vi "_Anritsu_SA_Write_Read.vi"(4 "bytes to read":i32=100, 6 "Comand":string="SNGLS\nSMA? 0,11", 7 "address":string="192.168.0.6") -> (0 "error out":errorcluster, 3 "Data out":i32[](array[numeric])=[-115184, -121571, -123353, -121687, -116570, -110499, -109976, -114455, -117677, -117596, -114322])   [LabVIEW 2013]
panel:
  out "data out":string="-115184,-121571,-123353,-121687,-116570,-110499,-109976,-114455,-117677,-117596,-114322\r\n"
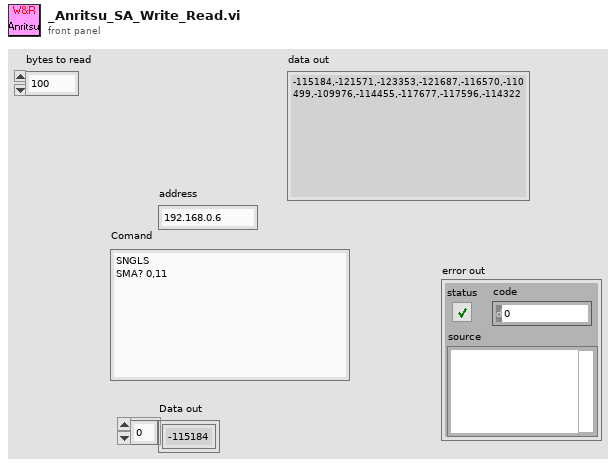
[diagram p1: front panel]
types:
  T1 = enum16{"Standard", "Buffered", "CRLF", "Immediate"}
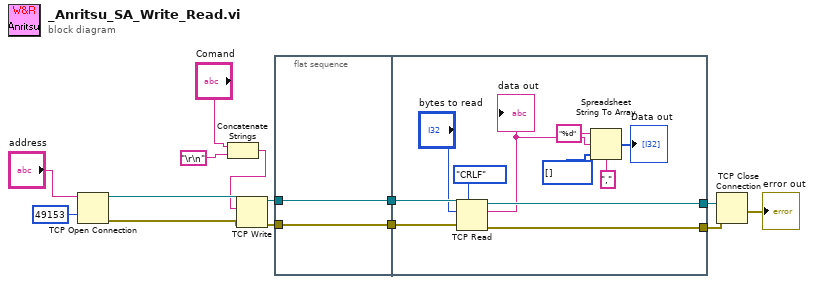
[diagram p0: block diagram]
diagram:
  n1 = TCP Open Connection(address="address", remote port or service name=u16 49153) -> (connection ID=w14:refnum<k5>, error out=w13:errorcluster)  [unwired: 3 in]
  n2 = Concatenate Strings("Comand", "\r\n") -> (w1:string)
  n3 = TCP Write(connection ID=w14, data in=w1, error in (no error)=w13) -> (connection ID out=w6:refnum<k5>, error out=w5:errorcluster)  [unwired: 1 in, 1 out]
  n4 = flat-sequence {
    tunnel: w5 -> [w15]
    tunnel: w6 -> [w16]
    tunnel: [w16] -> w4
    tunnel: [w15] -> w3
    tunnel: [w27] -> w9
    tunnel: [w26] -> w8
    tunnel: w4 -> [w25]
    tunnel: w3 -> [w24]
    frame #0 {
    }
    frame #1 {
      n5 = TCP Read(connection ID=w25, bytes to read="bytes to read", error in (no error)=w24, 7:T1."CRLF" ("mode (standard)")) -> (connection ID out=w27:refnum<k5>, data out=w19:string, error out=w26:errorcluster)  [unwired: 1 in]
      "data out" <- w19
      n6 = Spreadsheet String To Array(delimiter (Tab)=",", format string="%d", spreadsheet string=w19, array type (2D Dbl)=i32[] [] ("array")) -> (array=→"Data out":i32[])
    }
  }
  n7 = TCP Close Connection(connection ID=w9, error in (no error)=w8) -> (error out=→"error out":errorcluster)  [unwired: 1 in, 1 out]
